vi "DoInit.vi"(8 "error in (no error)":errorcluster, 11 "MainMenu in":refnum<class "MainMenu.lvclass">) -> (0 "error out":errorcluster, 3 "MainMenu out":refnum<class "MainMenu.lvclass">)   [LabVIEW 2019, in "RT_Game.lvlib" / "MainMenu.lvclass"]
uses:
  MainMenu.lvclass
  SnakeGame/SnakeGame.lvclass
  Pong/Pong.lvclass
  RT_Sprite/RT_Sprite.lvclass
  Game/Coordinate.ctl
  Bouncer/Bouncer.lvclass
  Menu/Menu.lvclass
  C:/Users/FreshBob/Dropbox/VIs/myRIO_GameConsole/RT/RT_Game/Game/Game.lvclass
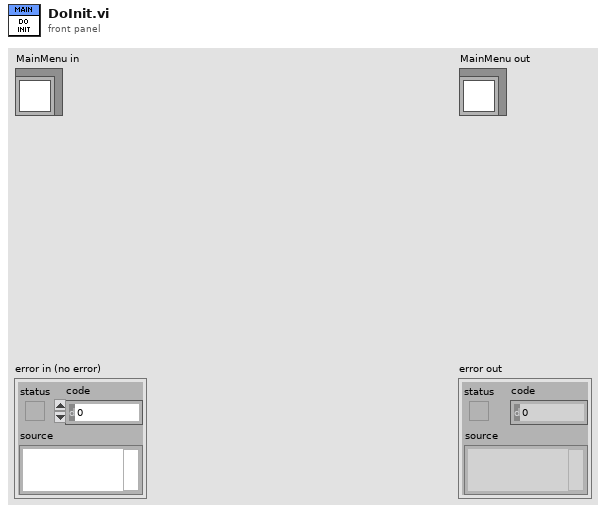
[diagram p1: front panel]
types:
  T1 = typedef "RT_Game.lvlib/Game.lvclass/Coordinate.ctl" = cluster{"x":dbl, "y":dbl}
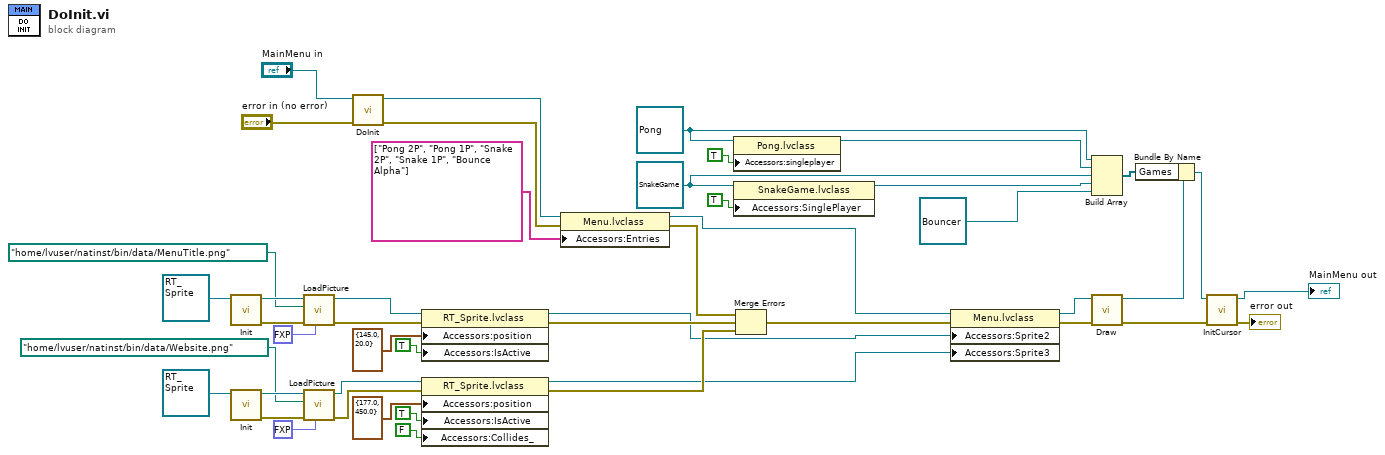
[diagram p0: block diagram]
diagram:
  w37 = refnum<class "Pong.lvclass"> refnum ("RT_Game.lvlib:Pong.lvclass")
  w35 = refnum<class "SnakeGame.lvclass"> refnum ("RT_Game.lvlib:Snake.lvclass")
  n1 = call-dynamic "Init.vi"("RT_Sprite in"=refnum<class "RT_Sprite.lvclass"> refnum ("RT_Game.lvlib:RT_Sprite.lvclass")) -> ("error out"=w31:errorcluster, "RT_Sprite out"=w32:refnum<class "RT_Sprite.lvclass">)  [unwired: 9 in]
  n2 = call-dynamic "Init.vi"("RT_Sprite in"=refnum<class "RT_Sprite.lvclass"> refnum ("RT_Game.lvlib:RT_Sprite.lvclass")) -> ("error out"=w20:errorcluster, "RT_Sprite out"=w21:refnum<class "RT_Sprite.lvclass">)  [unwired: 9 in]
  n3 = call "LoadPicture.vi"("Transparent Color"=fxp<+,3,3> 1.0, "error in (no error)"=w31, "Picture Path"=path "/home/lvuser/natinst/bin/data/MenuTitle.png", "RT_Sprite in"=w32) -> ("error out"=w28:errorcluster, "RT_Sprite out"=w29:refnum<class "RT_Sprite.lvclass">)  [unwired: 6 in]
  n4 = call "LoadPicture.vi"("Transparent Color"=fxp<+,3,3> 3.0, "error in (no error)"=w20, "Picture Path"=path "/home/lvuser/natinst/bin/data/Website.png", "RT_Sprite in"=w21) -> ("error out"=w17:errorcluster, "RT_Sprite out"=w18:refnum<class "RT_Sprite.lvclass">)  [unwired: 6 in]
  n5 = call-parent "DoInit.vi"("error in (no error)"="error in (no error)", "Menu in"="MainMenu in") -> ("error out"=w46:errorcluster, "Menu out"=w1:refnum<class "Menu.lvclass">)  [unwired: 8 in]
  n6 = property class="RT_Sprite.lvclass"(reference=w29, error in=w28, "Accessors:position"=T1 {"x"=145.0, "y"=20.0} ("position"), "Accessors:IsActive"=TRUE ("IsActive")) -> (reference out=w8:refnum<class "RT_Sprite.lvclass">, error out=w25:errorcluster)
  n7 = property class="RT_Sprite.lvclass"(reference=w18, error in=w17, "Accessors:position"=T1 {"x"=177.0, "y"=450.0} ("position"), "Accessors:IsActive"=TRUE ("IsActive"), "Accessors:Collides_"=FALSE ("Collides_")) -> (reference out=w7:refnum<class "RT_Sprite.lvclass">, error out=w12:errorcluster)
  n8 = property class="Menu.lvclass"(reference=w1, error in=w46, "Accessors:Entries"=string[] ["Pong 2P", "Pong 1P", "Snake 2P", "Snake 1P", "Bounce Alpha"] ("Entries")) -> (reference out=w10:refnum<class "Menu.lvclass">, error out=w42:errorcluster)
  n9 = property class="Pong.lvclass"(reference=w37, "Accessors:singleplayer"=TRUE ("singleplayer")) -> (reference out=w36:refnum<class "Pong.lvclass">)  [unwired: 1 in, 1 out]
  n10 = property class="SnakeGame.lvclass"(reference=w35, "Accessors:SinglePlayer"=TRUE ("SinglePlayer")) -> (reference out=w34:refnum<class "SnakeGame.lvclass">)  [unwired: 1 in, 1 out]
  n11 = Merge Errors(w42, w25, w12) -> (w26:errorcluster)
  n12 = property class="Menu.lvclass"(reference=w10, error in=w26, "Accessors:Sprite2"=w8, "Accessors:Sprite3"=w7) -> (reference out=w9:refnum<class "Menu.lvclass">, error out=w11:errorcluster)
  n13 = Build Array(w37, w36, w35, w34, refnum<class "Bouncer.lvclass"> refnum ("RT_Game.lvlib:Bouncer.lvclass")) -> (w2:refnum<class "Game.lvclass">[])
  n14 = call "Draw.vi"("error in (no error)"=w11, "Menu in"=w9) -> ("error out"=w40:errorcluster, "Menu out"=w39:refnum<class "MainMenu.lvclass">)  [unwired: 8 in]
  n15 = Bundle By Name(cluster=w39, "Games"=w2) -> (w5:refnum<class "MainMenu.lvclass">)
  n16 = call "InitCursor.vi"("error in (no error)"=w40, "Menu in"=w5) -> ("error out"=→"error out":errorcluster, "Menu out"=→"MainMenu out":refnum<class "MainMenu.lvclass">)  [unwired: 8 in]
